vi "setSenM.vi"(8 "error in (no error)":errorcluster, 9 "Sensitivity Matrix Shape":T1={"Num of Field"=35, "Num of Zk"=19, "Num of DOF"=50}, 10 "Sen M File Name":string="senM_35_19_50.txt", 11 "OptStateEsti in":refnum<class "OptStateEsti.lvclass">) -> (0 "error out":errorcluster, 3 "OptStateEsti out":refnum<class "OptStateEsti.lvclass">)   [LabVIEW 2016, in "OptStateEsti.lvclass"]
doc: "Set the sensitivity matrix M from file with the assigned index arrays of Zk and DOF."
uses:
  OptStateEsti.lvclass
  OptStateEsti.lvclass/OptStateEsti.ctl
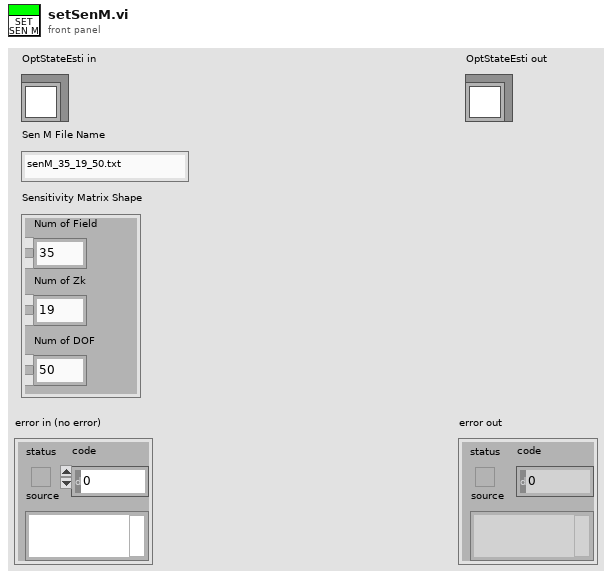
[diagram p1: front panel]
types:
  T1 = cluster{"Num of Field":i32, "Num of Zk":i32, "Num of DOF":i32}
  T2 = cluster{"Idx Array":i32[], "zn3Idx":i16[], "dofIdx":i16[]}
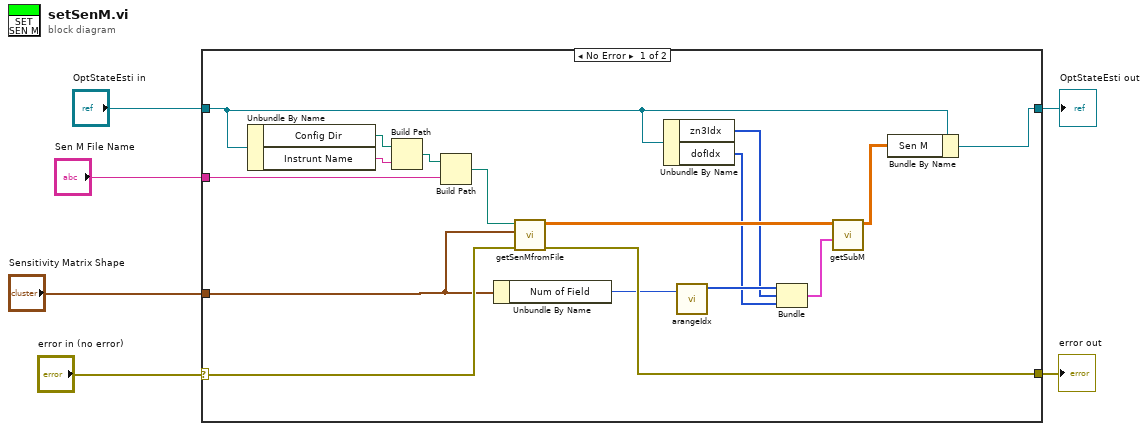
[diagram p0: block diagram]
diagram:
  n1 = case shown="No Error" "error in (no error)" {
    selector: "error in (no error)" -> [w23 w25]
    tunnel: [w22 w25] -> w5
    tunnel: [w13 w24] -> w3
    tunnel: "OptStateEsti in" -> [w7 w24]
    tunnel: "Sensitivity Matrix Shape" -> [w20 _]
    tunnel: "Sen M File Name" -> [w9 _]
    frame No Error {
      n2 = Unbundle By Name(w7) -> ("Config Dir"=w12:path, "Instrunt Name"=w11:string)
      n3 = Build Path(base path=w12, name or relative path=w11) -> (appended path=w10:path)
      n4 = Build Path(base path=w10, name or relative path=w9) -> (appended path=w8:path)
      n5 = Unbundle By Name(w20) -> ("Num of Field"=w19:i32)
      n6 = call "getSenMfromFile.vi"("error in"=w23, "Sensitivity Matrix Shape"=w20, "Path"=w8) -> ("error out"=w22:errorcluster, "Sensitivity Matrix"=w21:dbl[][][])  [unwired: 7 in]
      n7 = Unbundle By Name(w7) -> ("zn3Idx"=w17:i16[], "dofIdx"=w16:i16[])
      n8 = call "arangeIdx.vi"("Number"=w19) -> ("Idx Array"=w18:i32[])  [unwired: 10 in]
      n9 = Bundle("Idx Array"=w18, "zn3Idx"=w17, "dofIdx"=w16) -> (w15:T2)  [unwired: 1 in]
      n10 = call "getSubM.vi"("Index of Raws"=w15, "3D Matrix"=w21) -> ("Sub-Matrix"=w14:dbl[][][])  [unwired: 9 in]
      n11 = Bundle By Name(cluster=w7, "Sen M"=w14) -> (w13:refnum<class "OptStateEsti.lvclass">)
    }
    frame Error {
    }
  }
  "error out" <- w5
  "OptStateEsti out" <- w3
